vi "Cheksum Calculation Test.vi"(8 "Error In":errorcluster, 10 "Corrupted Message":T1={"Sender Name"="Test sender", "Recipent Name"="Test recipent", "Command"="Corruption", "Data"=variant, "Time Stamp"=timestamp(3755372400 s since 1904-01-01), "GUID"="1234", "Chcecksum"="4f781ef76083cfb2979f81dd45fbbf0e4be3ffcc552b5ace58ecc15638652f54"}, 11 "Correct Message":T1={"Sender Name"="Test sender", "Recipent Name"="Test recipent", "Command"="Test command", "Data"=variant, "Time Stamp"=timestamp(3755372400 s since 1904-01-01), "GUID"="1234", "Chcecksum"="4f781ef76083cfb2979f81dd45fbbf0e4be3ffcc552b5ace58ecc15638652f54"}) -> (0 "Error Out":errorcluster)   [LabVIEW 2023]
uses:
  Interfaces/ICanCommunicate/Message.ctl
  <vilib>/addons/_JKI Toolkits/Caraya/classes/Test/Test.lvclass
  Interfaces/ICanCommunicate/ICanCommunicate.lvclass
  <vilib>/addons/_JKI Toolkits/Caraya/classes/Assert/Assert.lvclass
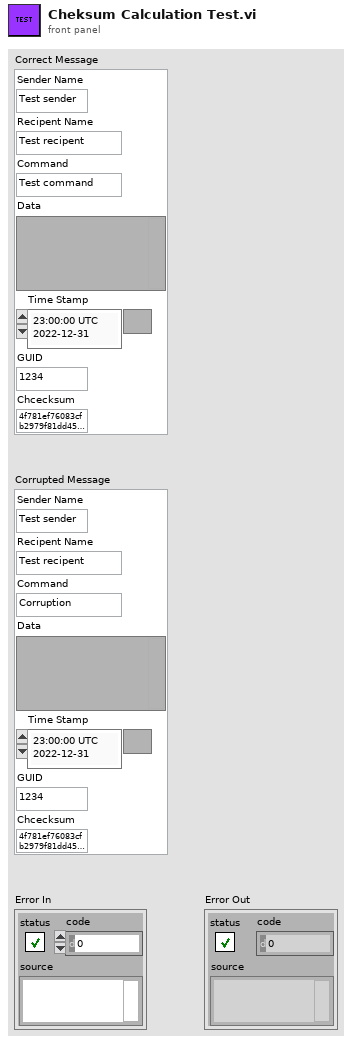
[diagram p1: front panel]
types:
  T1 = typedef "ICanCommunicate.lvclass/Message.ctl" = cluster{"Sender Name":string, "Recipent Name":string, "Command":string, "Data":variant, "Time Stamp":timestamp, "GUID":string, "Chcecksum":string}
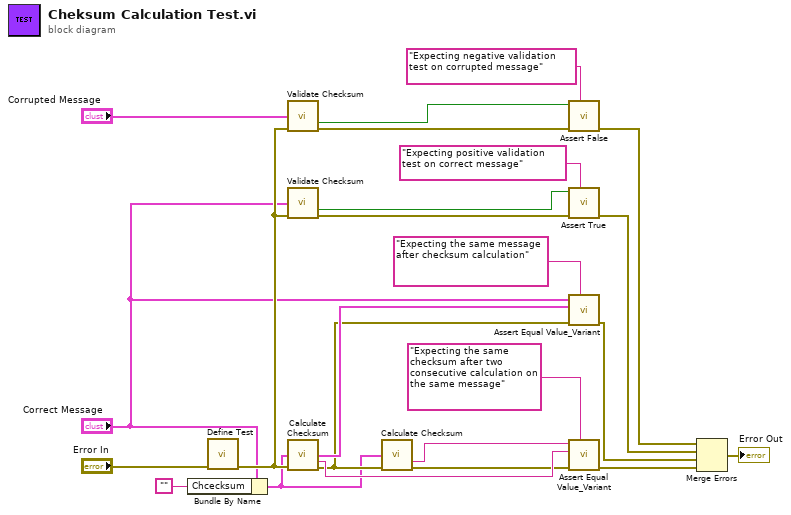
[diagram p0: block diagram]
diagram:
  n1 = Bundle By Name(cluster="Correct Message", "Chcecksum"="") -> (w1:T1)
  n2 = call <vilib>:"Define Test.vi"("error in (no error)"="Error In") -> ("error out"=w3:errorcluster)  [unwired: 9 in, 1 out]
  n3 = call "Validate Checksum.vi"("Message In"="Corrupted Message", "Error In"=w3) -> ("Valid?"=w20:bool, "Error Out"=w11:errorcluster)  [unwired: 11 in, 1 out]
  n4 = call "Validate Checksum.vi"("Message In"="Correct Message", "Error In"=w3) -> ("Valid?"=w21:bool, "Error Out"=w12:errorcluster)  [unwired: 11 in, 1 out]
  n5 = call "Calculate Checksum.vi"("Message In"=w1, "Error In"=w3) -> ("Message Out"=w18:T1, "Checksum"=w19:string, "Error Out"=w10:errorcluster)  [unwired: 11 in]
  n6 = call "Calculate Checksum.vi"("Message In"=w1, "Error In"=w10) -> ("Checksum"=w23:string, "Error Out"=w13:errorcluster)  [unwired: 11 in, 1 out]
  n7 = call <vilib>:"Assert False.vi"("Label"="Expecting negative validation test on corrupted message", "error in (no error)"=w11, "False?"=w20) -> ("error out"=w9:errorcluster)  [unwired: 7 in, 1 out]
  n8 = call <vilib>:"Assert True.vi"("Label"="Expecting positive validation test on correct message", "error in (no error)"=w12, "True?"=w21) -> ("error out"=w8:errorcluster)  [unwired: 7 in, 1 out]
  n9 = call <vilib>:"Assert Equal Value_Variant.vi"("Label"="Expecting the same message after checksum calculation", "error in (no error)"=w10, "Y"=w18, "X"="Correct Message") -> ("error out"=w7:errorcluster)  [unwired: 6 in, 1 out]
  n10 = call <vilib>:"Assert Equal Value_Variant.vi"("Label"="Expecting the same checksum after two consecutive calculation on the same message", "error in (no error)"=w13, "Y"=w19, "X"=w23) -> ("error out"=w6:errorcluster)  [unwired: 6 in, 1 out]
  n11 = Merge Errors(w9, w8, w7, w6) -> (→"Error Out":errorcluster)
